vi "cmdWithOptionalQueue.vi"(7 "LabVIEW Web Service Request":refnum<class "Web Request.lvclass">, 11 "queue":string) -> ()   [LabVIEW 2017]
uses:
  <vilib>/wsapi/Web Request.lvclass
  private/cmdSetup.ctl
  vsws_api/cmd.ctl
  vsws_api/vsws.lvlib
panel:
  # "Use the Web Service Request input terminal to call the VIs on the Web Services palette. Do not remove it from the connector pane unless you don't need access to the palette."
  # "Each additional control wired to the connector pane will be available as an input in the URL. To include an indicator in terminal-mode output (the default setting), it must also be wired to the connector pane."
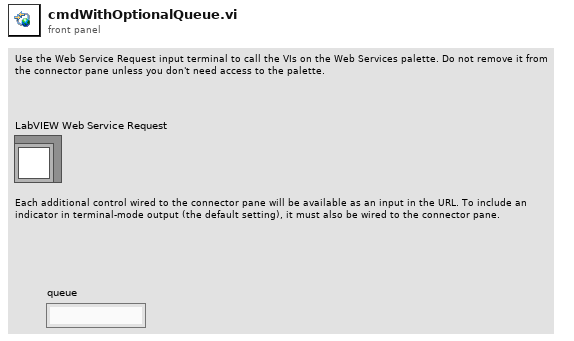
[diagram p1: front panel]
types:
  T1 = typedef "vsws.lvlib/cmd.ctl" = cluster{"postdata":string, "reponseQueue":refnum<queue>}
  T2 = typedef "cmdSetup.ctl" = cluster{"DefaultQueueName":string, "responseTimeout":i32, "logPostdata":string, "logResponse":string}
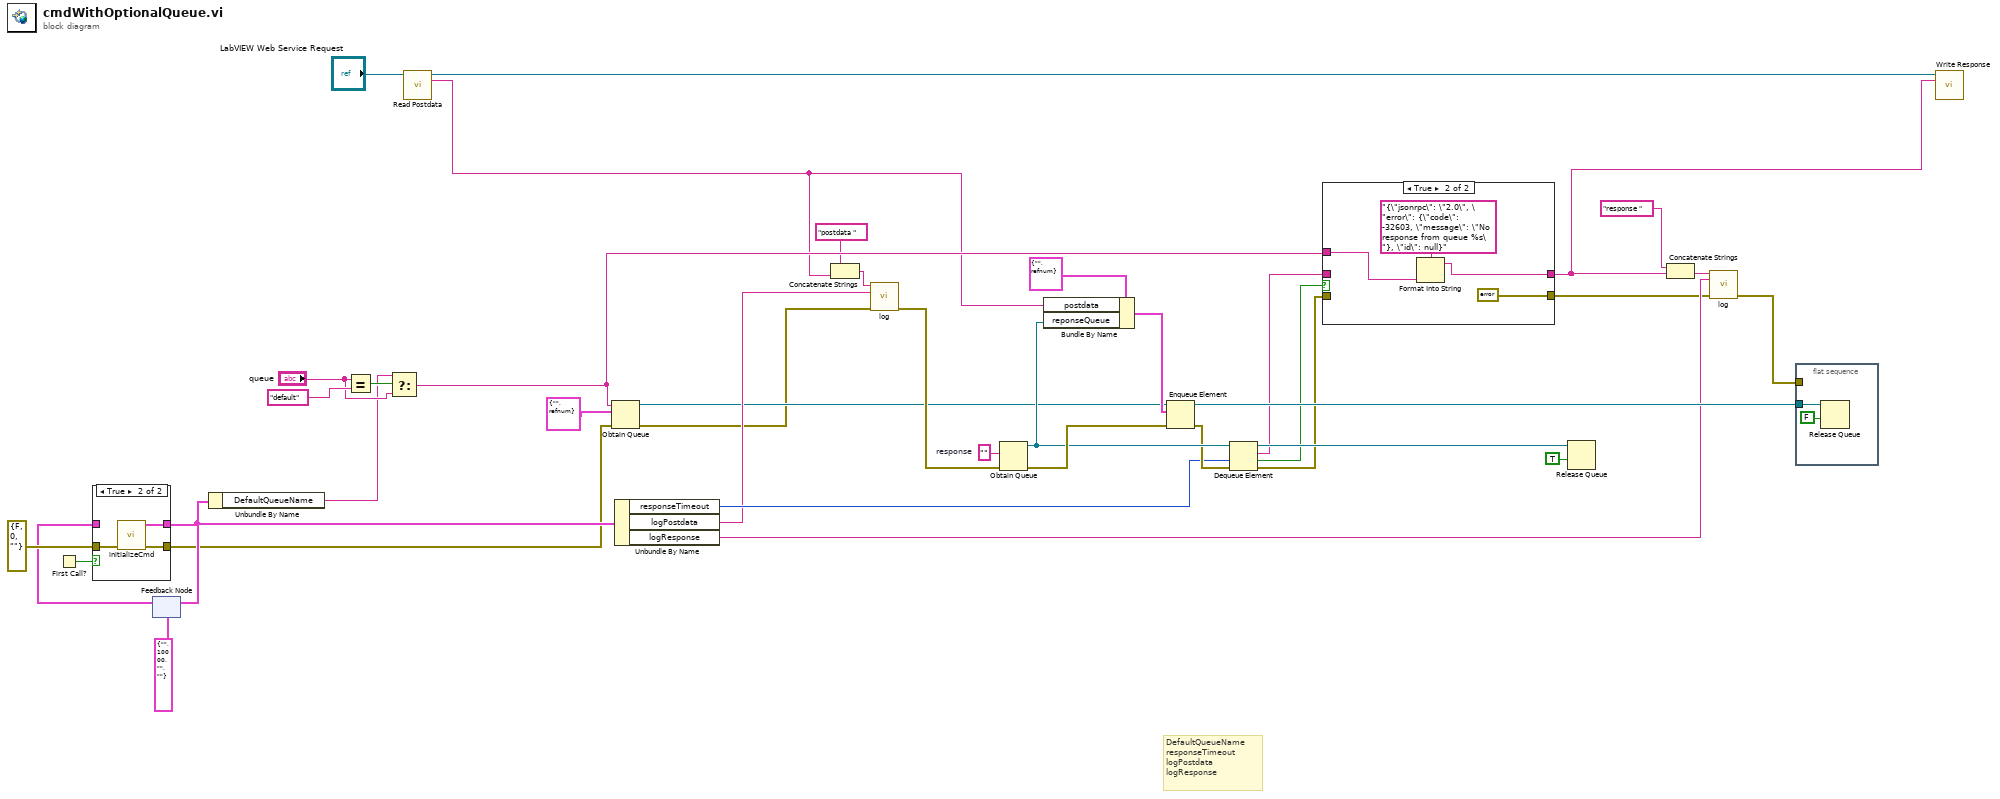
[diagram p0: block diagram]
diagram:
  w25 = ""  # response
  # "DefaultQueueName\nresponseTimeout\nlogPostdata\nlogResponse"
  n1 = First Call?() -> (First Call?: T/F=w39:bool)
  n2 = feedback #1(T2 {"DefaultQueueName"="", "responseTimeout"=10000, "logPostdata"="", "logResponse"=""} ("cmdSetup")) -> (w37:T2)
  n3 = case shown="True" w39 {
    tunnel: [w41 w43] -> w33
    tunnel: errorcluster {"status"=FALSE, "code"=0, "source"=""} ("error in (no error)") -> [w42 w45]
    tunnel: [w42 w44] -> w28
    tunnel: w37 -> [w41 _]
    frame False {
    }
    frame True {
      n4 = call "initializeCmd.vi"("error in (no error)"=w45) -> ("cmdSetup"=w43:T2, "error out"=w44:errorcluster)  [unwired: 13 in]
    }
  }
  n5 = feedback-in #1(w33) -> ()
  n6 = Unbundle By Name(w33) -> ("DefaultQueueName"=w32:string)
  n7 = Equal?(x="queue", y="default") -> (x = y?=w35:bool)
  n8 = Select(t=w32, s=w35, f="queue") -> (s? t:f=w31:string)
  n9 = call <vilib>:"Read Postdata.vi"("LabVIEW Web Service Request"="LabVIEW Web Service Request") -> ("LabVIEW Web Service Request out"=w26:refnum<class "Web Request.lvclass">, "postdata"=w29:string)  [unwired: 12 in, 1 out]
  n10 = Obtain Queue(name (unnamed)=w31, element data type=T1 {"postdata"="", "reponseQueue"=refnum} ("cmd"), error in (no error)=w28) -> (queue out=w14:refnum<queue>, error out=w1:errorcluster)  [unwired: 2 in, 1 out]
  n11 = Unbundle By Name(w33) -> ("responseTimeout"=w18:i32, "logPostdata"=w17:string, "logResponse"=w7:string)
  n12 = Concatenate Strings("postdata " ("string"), w29) -> (w11:string)
  n13 = call "log.vi"("log string"=w11, "logOption"=w17, "error in (no error)"=w1) -> ("error out"=w16:errorcluster)  [unwired: 12 in]
  n14 = Obtain Queue(element data type=w25, error in (no error)=w16) -> (queue out=w21:refnum<queue>, error out=w22:errorcluster)  [unwired: 3 in, 1 out]
  n15 = Bundle By Name(cluster=T1 {"postdata"="", "reponseQueue"=refnum} ("cmd"), "postdata"=w29, "reponseQueue"=w21) -> (w23:T1)
  n16 = Enqueue Element(queue=w14, element=w23, error in (no error)=w22) -> (queue out=w12:refnum<queue>, error out=w20:errorcluster)  [unwired: 1 in, 1 out]
  n17 = Dequeue Element(queue=w21, timeout in ms (-1)=w18, error in (no error)=w20) -> (queue out=w19:refnum<queue>, element=w2:string, timed out?=w5:bool, error out=w4:errorcluster)
  n18 = case shown="True" w5 {
    tunnel: w4 -> [w47 _]
    tunnel: [w47 errorcluster {"status"=FALSE, "code"=0, "source"=""} ("error out")] -> w3
    tunnel: w2 -> [w46 _]
    tunnel: [w46 w48] -> w27
    tunnel: w31 -> [_ w49]
    frame False {
    }
    frame True {
      n19 = Format Into String(format string="{\"jsonrpc\": \"2.0\", \"error\": {\"code\": -32603, \"message\": \"No response from queue %s\"}, \"id\": null}" ("response"), w49) -> (resulting string=w48:string)  [unwired: 2 in, 1 out]
    }
  }
  n20 = Release Queue(queue=w19, force destroy? (F)=TRUE) -> ()  [unwired: 1 in, 3 out]
  n21 = Concatenate Strings("response ", w27) -> (w8:string)
  n22 = call "log.vi"("log string"=w8, "logOption"=w7, "error in (no error)"=w3) -> ("error out"=w6:errorcluster)  [unwired: 12 in]
  n23 = flat-sequence {
    tunnel: w12 -> [w53]
    tunnel: w6 -> [_]
    frame #0 {
      n24 = Release Queue(queue=w53, force destroy? (F)=FALSE) -> ()  [unwired: 1 in, 3 out]
    }
  }
  n25 = call <vilib>:"Write Response.vi"("LabVIEW Web Service Request"=w26, "response string"=w27) -> ()  [unwired: 12 in, 2 out]
